vi "uBroker_Fanout.vi"(9 "uMsg":refnum<class "uMsg.lvclass">, 10 "uPub":refnum<class "uClient_Publisher.lvclass">, 11 "Cluster in":T2) -> (3 "Cluster out":T2)   [LabVIEW 2023, in "uLib.lvlib" / "uBroker.lvclass"]
uses:
  uBroker.lvclass
  TypeDef_uBrokerTopic.ctl
  uMsg/uMsg/uMsg.lvclass
  uClient/uClient_Publisher/uClient_Publisher.lvclass
  uSubscription/uSubscription/uSubscription.lvclass
  uClient/uClient_Subscriber/uClient_Subscriber.lvclass
  U:/Projects/uLib/Src/uFramework/uClient/uClient.lvclass
  uMsg/uMsg/uMsg.lvclass/uMsg.ctl
  <vilib>/Utility/miscctls.llb/LVMapReplaceAction.ctl
  uClient/uClient_Publisher/uClient_Publisher.lvclass/uClient_Publisher.ctl
  uClient/uClient/uClient.lvclass/uClient.ctl
  uClient/uClient_Subscriber/uClient_Subscriber.lvclass/uClient_Subscriber.ctl
  uPolicy/uPolicy/uPolicy.lvclass/uPolicy.ctl
  uSubscription/uSubscription/uSubscription.lvclass/uSubscription.ctl
  uNotifyMode/uNotifyMode/uNotifyMode.lvclass/uNotifyMode.ctl
  uTransport/uTransport_uActor/uTransport_uActor.lvclass/uTransport_uActor.ctl
  uTransport/uTransport_Event/uTransport_Event.lvclass/uTransport_Event.ctl
  uTransport/uTransport_Queue/uTransport_Queue.lvclass/uTransport_Queue.ctl
  uMsg/uMsg/uMsg Rename CMD.vi
  uNotifyMode/uNotifyMode/uNotify Update.vi
  uClient/uClient/uClient_GetTransport.vi
  uClient/uClient_Subscriber/uSubscriber Get uPolicy.vi
  uPolicy/uPolicy/Read uNotifyMode.vi
  uPolicy/uPolicy/Read uStringManipulation.vi
  uTransport/uTransport/uTransport_SendMsg.vi
  uTransport/uTransport_uActor/uTransport_uActor_SendMsg.vi
  uTransport/uTransport_Event/uTransport_Event_SendMsg.vi
  uTransport/uTransport_Queue/uTransport_Queue_SendMsg.vi
  uMsg/uMsg/uMsg Update Timestamp.vi
  uNotifyMode/uNotifyMode/uNotifyMode.lvclass
  uTransport/uTransport/uTransport.lvclass
  uPolicy/uPolicy/uPolicy.lvclass
  uStringManipulation/uStringManipulation/uStringManipulation.lvclass
  uTransport/uTransport_uActor/uTransport_uActor.lvclass
  uTransport/uTransport_Event/uTransport_Event.lvclass
  uTransport/uTransport_Queue/uTransport_Queue.lvclass
  uBroker.lvclass/uBroker.ctl
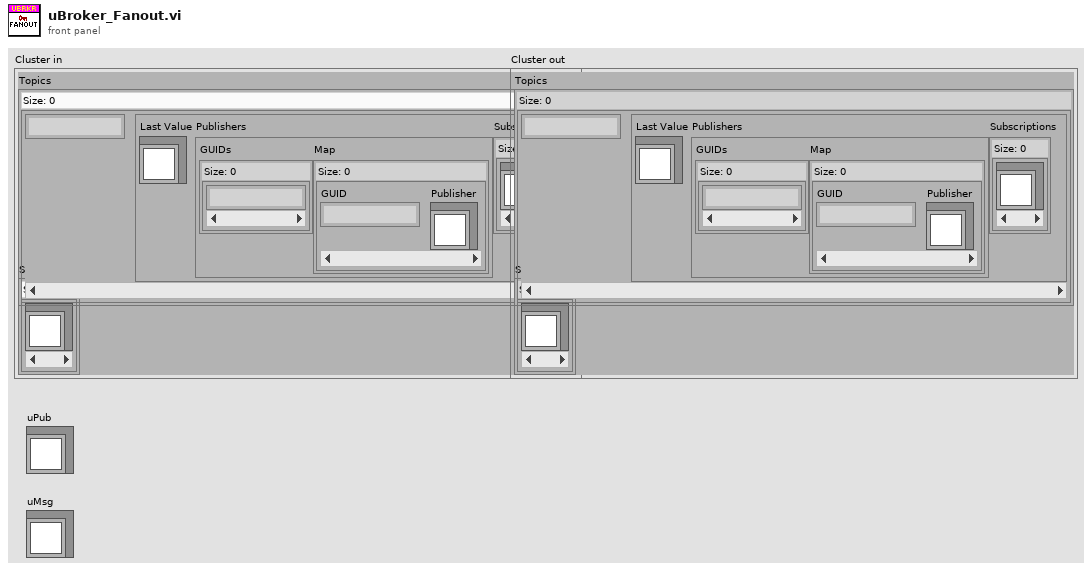
[diagram p1: front panel]
types:
  T1 = typedef "uLib.lvlib/uBroker.lvclass/TypeDef_uBrokerTopic.ctl" = cluster{"Last Value":refnum<class "uMsg.lvclass">, "Publishers":cluster{"GUIDs":set{string}, "Map":map{string, refnum<class "uClient_Publisher.lvclass">}}, "Subscriptions":set{refnum<class "uSubscription.lvclass">}}
  T2 = cluster{"Topics":map{string, T1}, "Subscribers":set{refnum<class "uClient_Subscriber.lvclass">}}
  T3 = typedef "LVMapReplaceAction.ctl" = enum32{"Modify Entry only if found", "Add or Modify Entry", "Delete Entry"}
  T4 = map{string, refnum<class "uClient_Publisher.lvclass">}
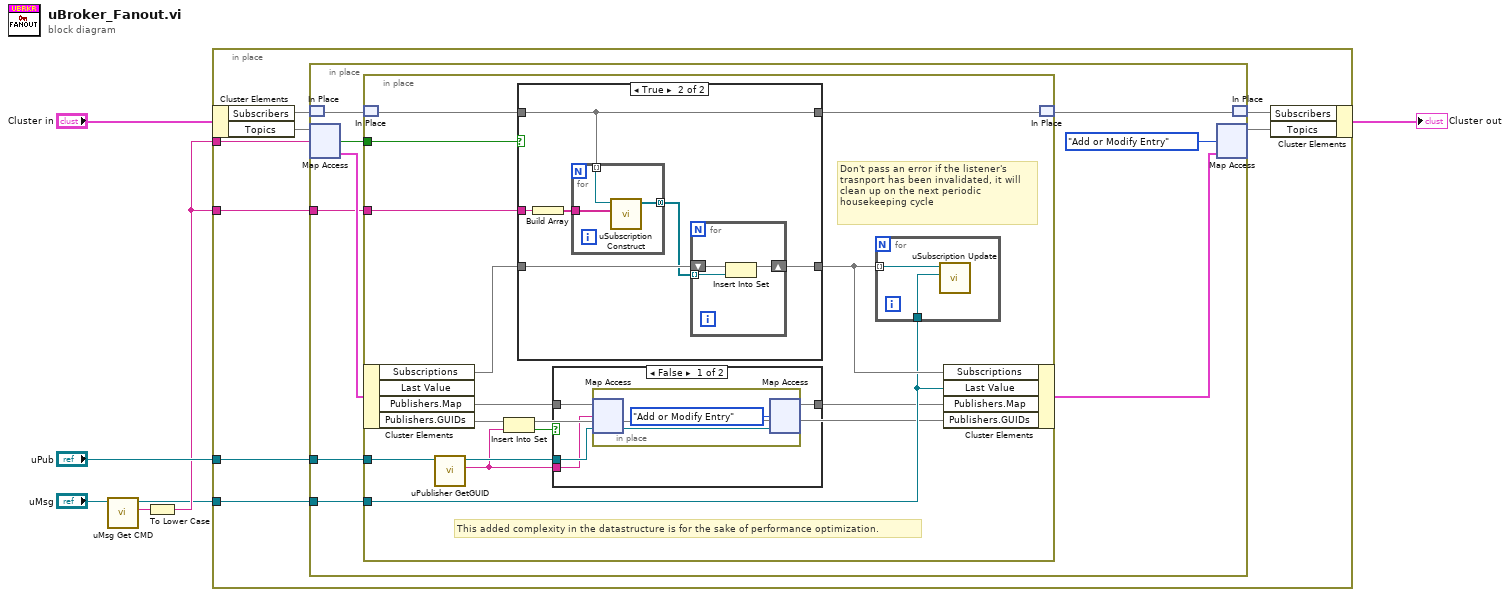
[diagram p0: block diagram]
diagram:
  n1 = call "uMsg Get CMD.vi"("uMsg in"="uMsg") -> ("CMD"=w2:string, "uMsg out"=w3:refnum<class "uMsg.lvclass">)  [unwired: 8 in, 1 out]
  n2 = To Lower Case(string=w2) -> (all lower case string=w4:string)
  n3 = in-place {
    in-place-border: w4 -> [w12]
    in-place-border: w3 -> [w13]
    in-place-border: "uPub" -> [w11]
    in-place-border: w4 -> [w10]
    n4 = in-place-cluster #1("Cluster in") -> ("Subscribers"=w9:set{refnum<class "uClient_Subscriber.lvclass">}, "Topics"=w15:map{string, T1})
    n5 = in-place {
      in-place-border: w13 -> [w23]
      in-place-border: w11 -> [w22]
      in-place-border: w10 -> [w18]
      n6 = in-place-match #2(w9) -> (w16:set{refnum<class "uClient_Subscriber.lvclass">})
      n7 = in-place-map #3(w15, w12) -> (w20:T1, w21:bool)  [unwired: 1 in]
      n8 = in-place {
        in-place-border: w23 -> [w33]
        in-place-border: w22 -> [w32]
        in-place-border: w21 -> [w39]
        in-place-border: w18 -> [w36]
        # "This added complexity in the datastructure is for the sake of performance optimization."
        # "Don't pass an error if the listener's trasnport has been invalidated, it will clean up on the next periodic housekeeping cycle"
        n9 = in-place-match #4(w16) -> (w35:set{refnum<class "uClient_Subscriber.lvclass">})
        n10 = in-place-cluster #5(w20) -> ("Subscriptions"=w38:set{refnum<class "uSubscription.lvclass">}, "Publishers.Map"=w30:T4, "Publishers.GUIDs"=w28:set{string})  [unwired: 1 out]
        n11 = call "uPublisher GetGUID.vi"("uClient_Publisher in"=w32) -> ("GUID"=w27:string, "uClient_Publisher out"=w29:refnum<class "uClient_Publisher.lvclass">)  [unwired: 8 in, 1 out]
        n12 = Insert Into Set(10:w27, 11:w28) -> (2:w26:bool, 3:w25:set{string})
        n13 = case shown="True" w39 {
          tunnel: [w48 w54] -> w37
          tunnel: w38 -> [w48 w51]
          tunnel: w36 -> [_ w53]
          tunnel: w35 -> [w47 w49]
          tunnel: [w47 w49] -> w34
          frame False {
          }
          frame True {
            n14 = Build Array(w53) -> (w52:string[])
            n15 = for {
              tunnel: [w57] -> w50 mode=concatenating
              tunnel: w52 -> [w56]
              tunnel: w49 -> [w55] mode=indexing
              n16 = call "uSubscription Construct.vi"("Topics"=w56, "uClient_Subscriber"=w55) -> ("uSubscriptions out"=w57:refnum<class "uSubscription.lvclass">[])  [unwired: 7 in, 2 out]
            }
            n17 = for {
              shift-right: [w60] -> w54
              shift-left: w51 -> [w59]
              tunnel: w50 -> [w58] mode=indexing
              n18 = Insert Into Set(10:w58, 11:w59) -> (3:w60:set{refnum<class "uSubscription.lvclass">})  [unwired: 1 out]
            }
          }
        }
        n19 = case shown="False" w26 {
          tunnel: [w42 w46] -> w31
          tunnel: w30 -> [w43 w46]
          tunnel: w27 -> [w40 _]
          tunnel: w29 -> [w41 _]
          frame False {
            n20 = in-place {
              n21 = in-place-map #6(w43, w40, w41) -> (w44:refnum<class "uClient_Publisher.lvclass">)  [unwired: 1 out]
              n22 = in-place-map #6(w44, LVMapReplaceAction."Add or Modify Entry" ("action")) -> (w42:T4)  [unwired: 2 out]
            }
          }
          frame True {
          }
        }
        n23 = for {
          tunnel: w37 -> [w62] mode=indexing
          tunnel: w33 -> [w61]
          n24 = call "uSubscription Update.vi"("uMsg"=w61, "uSubscription in"=w62) -> ()  [unwired: 9 in, 1 out]
        }
        n25 = in-place-cluster #5("Subscriptions"=w37, "Last Value"=w33, "Publishers.Map"=w31, "Publishers.GUIDs"=w25) -> (w19:T1)
        n26 = in-place-match #4(w34) -> (w17:set{refnum<class "uClient_Subscriber.lvclass">})
      }
      n27 = in-place-map #3(w19, LVMapReplaceAction."Add or Modify Entry" ("action")) -> (w14:map{string, T1})  [unwired: 2 out]
      n28 = in-place-match #2(w17) -> (w8:set{refnum<class "uClient_Subscriber.lvclass">})
    }
    n29 = in-place-cluster #1("Subscribers"=w8, "Topics"=w14) -> (→"Cluster out":T2)
  }
